vi "buffer data.vi"(4 "Samples/second":dbl, 6 "buffer time (s)":dbl, 8 "error in":errorcluster, 9 "Data to write":sgl[](array[numeric]), 11 "task ID":T1 format="%.0x") -> (0 "error out":errorcluster, 3 "task ID out":T1 format="%.0x")   [LabVIEW 2009]
uses:
  <vilib>/sound2/lvsound2.llb/Sound Output Task ID.ctl
  <vilib>/sound2/lvsound2.llb/Sound Output Write (DBL Single).vi
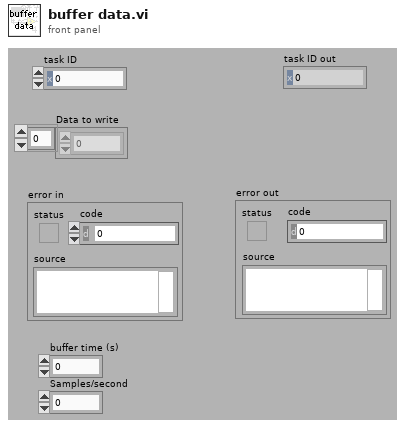
[diagram p1: front panel]
types:
  T1 = typedef "Sound Output Task ID.ctl" = u32
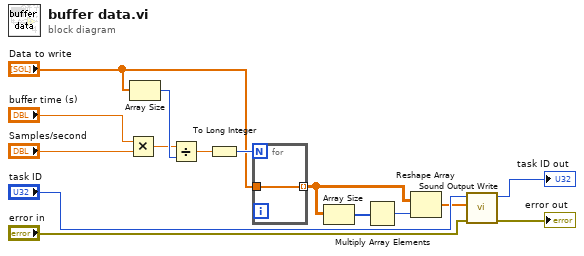
[diagram p0: block diagram]
diagram:
  n1 = Multiply(x="buffer time (s)", y="Samples/second") -> (x*y=w8:dbl)
  n2 = Array Size(array="Data to write") -> (size(s)=w9:i32)
  n3 = Divide(x=w8, y=w9) -> (x/y=w7:dbl)
  n4 = To Long Integer(number=w7) -> (32bit integer=w6:i32)
  n5 = for {
    N: w6 -> [_]
    tunnel: "Data to write" -> [w16]
    tunnel: [w16] -> w4 mode=indexing
  }
  n6 = Array Size(array=w4) -> (size(s)=w3:i32[])
  n7 = Multiply Array Elements(1:w3) -> (0:w2:i32)
  n8 = Reshape Array(w4, w2) -> (w1:sgl[])
  n9 = call-poly <vilib>:"Sound Output Write.vi"("error in (no error)"="error in", "data"=w1, "task ID"="task ID") -> ("error out"=→"error out":errorcluster, "task ID out"=→"task ID out":T1)  [unwired: 7 in]
